vi "popularVideos.vi"(8 "error in (no error)":errorcluster, 11 "YoutubeCacheProxy in":refnum<class "YoutubeCacheProxy.lvclass">) -> (0 "error out":errorcluster, 2 "cachePopular":T1, 3 "YoutubeCacheProxy out":refnum<class "YoutubeCacheProxy.lvclass">)   [LabVIEW 2017, in "YoutubeCacheProxy.lvclass"]
uses:
  YoutubeCacheProxy.lvclass
  Globals/HashMap.ctl
  Video Class/Video.lvclass
  YoutubeCacheProxy.lvclass/YoutubeCacheProxy.ctl
  ThirdPartyYoutubeLib Class/ThirdPartyYoutubeLib.lvclass
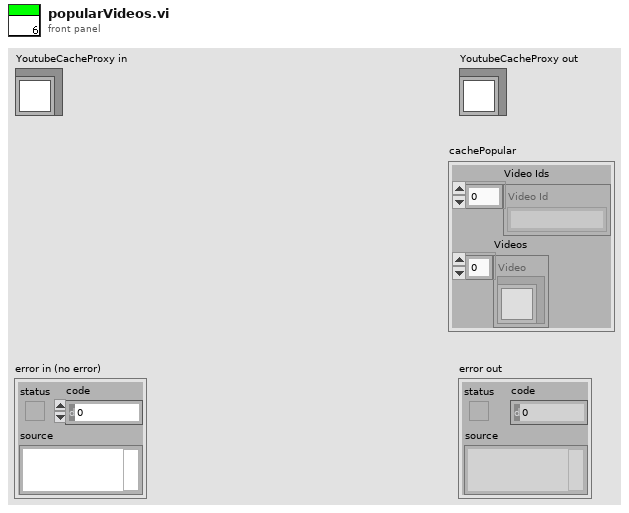
[diagram p1: front panel]
types:
  T1 = typedef "HashMap.ctl" = cluster{"Video Ids":string[], "Videos":refnum<class "Video.lvclass">[]}
  T2 = enum16{"Create", "Get Reference", "Print", "Close"}
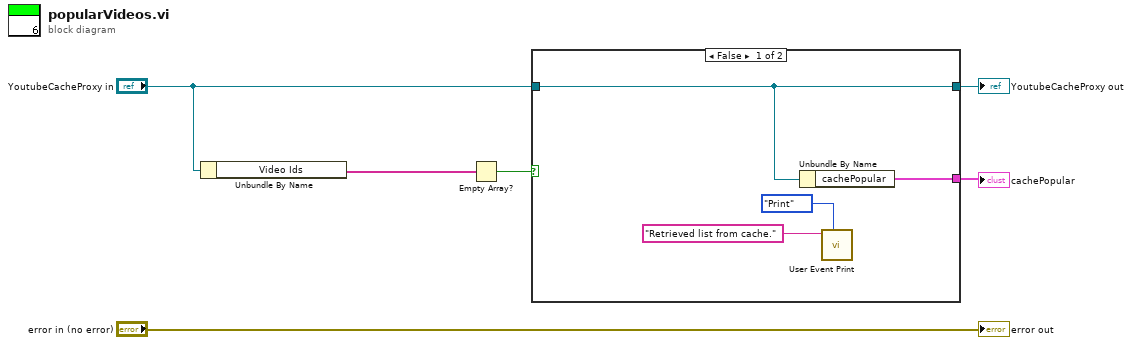
[diagram p0: block diagram]
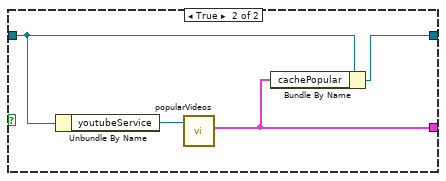
[diagram p2: hidden frame]
diagram:
  n1 = Unbundle By Name("YoutubeCacheProxy in") -> ("Video Ids"=w5:string[])
  n2 = Empty Array?(array=w5) -> (empty?=w4:bool)
  n3 = case shown="False" w4 {
    tunnel: "YoutubeCacheProxy in" -> [w10 w14]
    tunnel: [w10 w12] -> w2
    tunnel: [w9 w11] -> w1
    frame False {
      n4 = Unbundle By Name(w10) -> ("cachePopular"=w9:T1)
      n5 = call "User Event Print.vi"("Options"=T2."Print", "String to Print"="Retrieved list from cache." ("ConsoleOut")) -> ()  [unwired: 8 in, 2 out]
    }
    frame True {
      n6 = Unbundle By Name(w14) -> ("youtubeService"=w13:refnum<class "ThirdPartyYoutubeLib.lvclass">)
      n7 = call-dynamic "popularVideos.vi"("ThirdPartyYoutubeLib in"=w13) -> ("HashMap"=w11:T1)  [unwired: 8 in, 2 out]
      n8 = Bundle By Name(cluster=w14, "cachePopular"=w11) -> (w12:refnum<class "YoutubeCacheProxy.lvclass">)
    }
  }
  "YoutubeCacheProxy out" <- w2
  "cachePopular" <- w1
  "error out" <- "error in (no error)"
